vi "Data from Channel 0.vi"() -> (3 "Channel Data":i16[](array[numeric]))   [LabVIEW 2012]
uses:
  <vilib>/rvi/eio/common/nirviEmuTemplateMethod_errors.vi
  <vilib>/eio/EIONode/EIONode.xnode
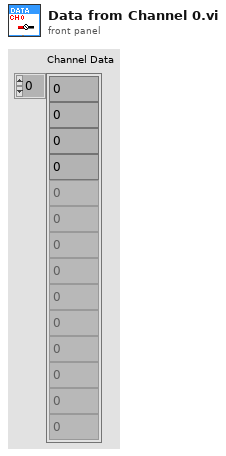
[diagram p1: front panel]
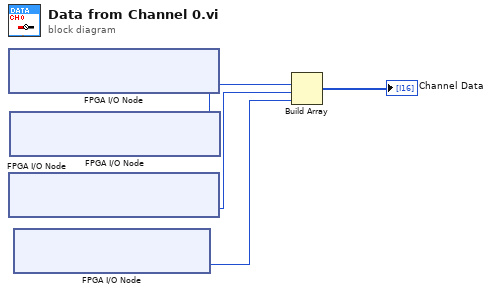
[diagram p0: block diagram]
diagram:
  n1 = xnode "FPGA I/O Node"() -> ("IO Module\\AI 0 Data N-3"=w5:i16)  [unwired: 1 in, 1 out]
  n2 = xnode "FPGA I/O Node"() -> ("IO Module\\AI 0 Data N-1"=w2:i16)  [unwired: 1 in, 1 out]
  n3 = xnode "FPGA I/O Node"() -> ("IO Module\\AI 0 Data N-2"=w3:i16)  [unwired: 1 in, 1 out]
  n4 = xnode "FPGA I/O Node"() -> ("IO Module\\AI 0 Data N"=w1:i16)  [unwired: 1 in, 1 out]
  n5 = Build Array(w5, w3, w2, w1) -> (→"Channel Data":i16[])
